vi "Amplitud.vi"(8 "error in (no error)":errorcluster, 10 "Amplitud":dbl, 11 "Measurement gg in":refnum<class "Measurement gg.lvclass">) -> (0 "error out":errorcluster, 3 "Measurement gg out":refnum<class "Measurement gg.lvclass">)   [LabVIEW 2020, in "Measurement gg.lvlib" / "Measurement gg.lvclass"]
uses:
  Measurement gg.lvclass
  Measurement gg.lvclass/Measurement gg.ctl
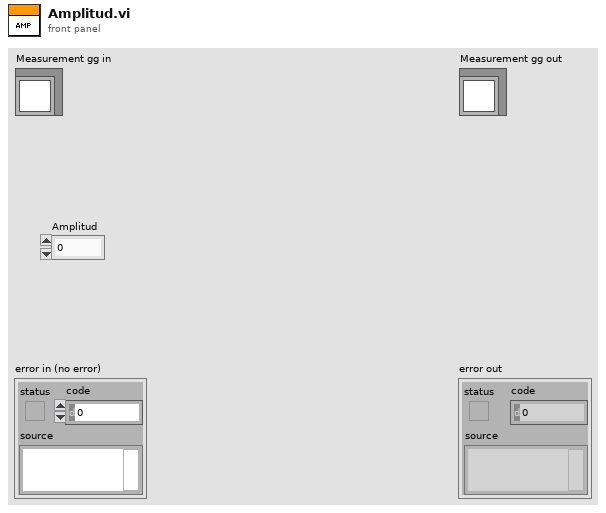
[diagram p1: front panel]
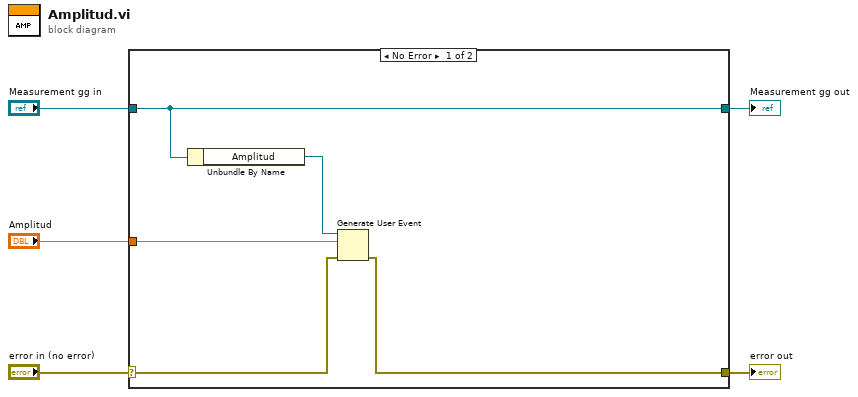
[diagram p0: block diagram]
diagram:
  n1 = case shown="No Error" "error in (no error)" {
    selector: "error in (no error)" -> [w10 w12]
    tunnel: [w9 w12] -> w4
    tunnel: [w8 w11] -> w2
    tunnel: "Measurement gg in" -> [w8 w11]
    tunnel: "Amplitud" -> [w6 _]
    frame No Error {
      n2 = Unbundle By Name(w8) -> ("Amplitud"=w7:refnum<user-event>)
      n3 = Generate User Event(user event=w7, event data cluster=w6, error in=w10) -> (error out=w9:errorcluster)  [unwired: 1 in, 1 out]
    }
    frame Error {
    }
  }
  "error out" <- w4
  "Measurement gg out" <- w2
